vi "Search Error Codes.vi"(7 "searched objects":i32[](array[numeric]), 11 "scope error codes":i32[](array[numeric])) -> (3 "found codes indices":i32[](array[numeric]))   [LabVIEW 2017]
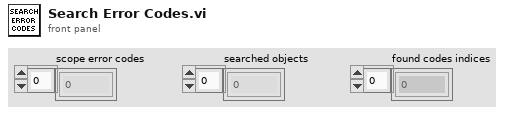
[diagram p1: front panel]
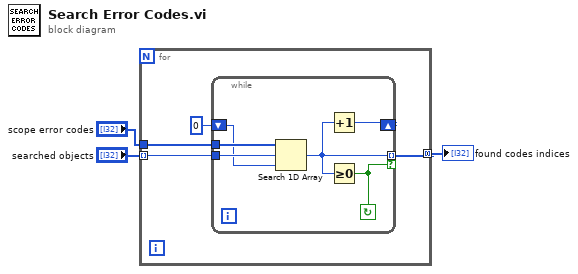
[diagram p0: block diagram]
diagram:
  n1 = for {
    tunnel: "scope error codes" -> [w7]
    tunnel: [w6] -> w2 mode=concatenating
    tunnel: "searched objects" -> [w4] mode=indexing
    n2 = while {
      tunnel: w4 -> [w12]
      tunnel: w7 -> [w13]
      tunnel: [w10] -> w6 mode=indexing if=w11
      shift-right: [w9] -> _
      shift-left: 0 -> [w8]
      stop <- w11 continue-if-true
      n3 = Search 1D Array(1D array=w13, element=w12, start index (0)=w8) -> (index of element=w10:i32)
      n4 = Increment(x=w10) -> (x+1=w9:i32)
      n5 = Greater Or Equal To 0?(x=w10) -> (x >= 0?=w11:bool)
    }
  }
  "found codes indices" <- w2
